vi "CreateBarCode.vi"(8 "error in (no error)":errorcluster, 10 "Input":string, 11 "BarCode in":refnum<class "BarCode.lvclass">) -> (0 "error out":errorcluster, 1 "Valid Value":bool, 2 "Barcode":picture, 3 "BarCode out":refnum<class "BarCode.lvclass">)   [LabVIEW 2013, in "BarCodes.lvlib" / "BarCode.lvclass"]
doc: "Creates a bar code to represent the specified text. If the text cannot be represented as a bar code in the format defined by this class, Valid Value will return false."
uses:
  BarCode.lvclass
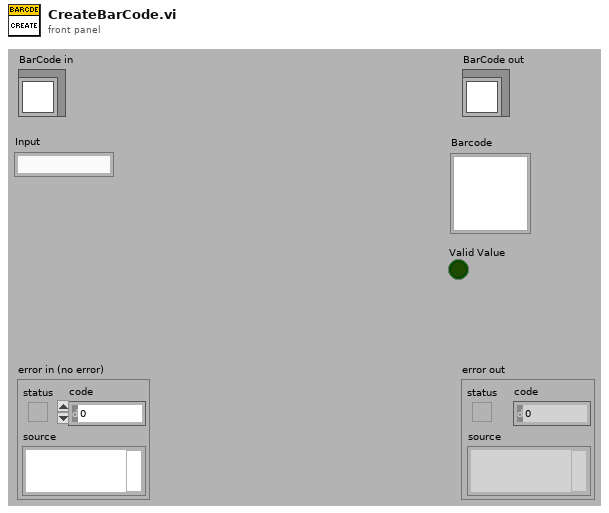
[diagram p1: front panel]
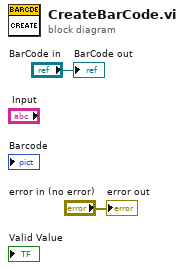
[diagram p0: block diagram]
diagram:
  "error out" <- "error in (no error)"
  "BarCode out" <- "BarCode in"
